vi "SetIOPinSignalMode.vi"(8 "错误输入（无错误）":errorcluster, 9 "信号模式":u8) -> (0 "错误输出":errorcluster)   [LabVIEW 2014]
uses:
  X86Dll/ZXUTConfigMgr.dll
panel:
  in  "SelPinType":i32
  in  "SelPinNum":i32
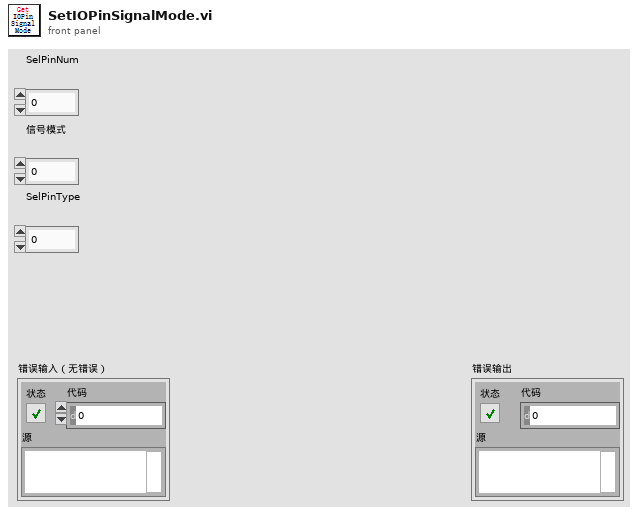
[diagram p1: front panel]
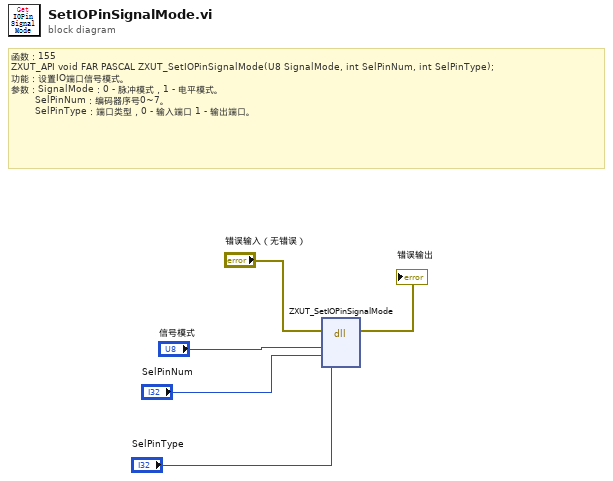
[diagram p0: block diagram]
diagram:
  # "函数：155\nZXUT_API void\tFAR PASCAL ZXUT_SetIOPinSignalMode(U8 SignalMode, int SelPinNum, int SelPinType);\n功能：设置IO端口信号模式。\n参数：SignalMode：0 - 脉冲模式，1 - 电平模式。\n        SelPinNum：编码器序号0~7。\n        SelPinType：端口类型，0 - 输入端口 1 - 输出端口。"
  n1 = dll-call lib="D:/Software/Utrasonic on-line monitoring/X86Dll/ZXUTConfigMgr.dll" fn="ZXUT_SetIOPinSignalMode"(error in="错误输入（无错误）", "SignalMode"="信号模式", "SelPinNum"="SelPinNum", "SelPinType"="SelPinType") -> (error out=→"错误输出":errorcluster)  [unwired: 6 in, 1 out]
